vi "Rotate.vi"(8 "error in":errorcluster, 9 "Inverse?":bool, 10 "Orient3d in":refnum<class "Orient3d Class.lvclass">, 11 "Vec3d in":refnum<class "Vec3d Class.lvclass">) -> (0 "error out":errorcluster, 3 "Vec3d out":refnum<class "Vec3d Class.lvclass">)   [LabVIEW 2011, in "Vec3d Class.lvclass"]
uses:
  Vec3d Class.lvclass
  Orient3d Class/Orient3d Class.lvclass
  Vec3d Class.lvclass/Vec3d Class.ctl
  <vilib>/Analysis/baseanly.llb/Real A x B.vi
  <vilib>/Analysis/NI_AALBase.lvlib
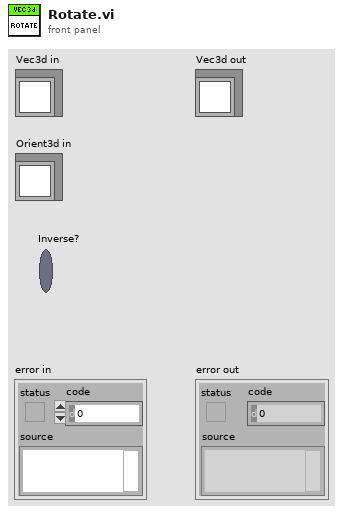
[diagram p1: front panel]
types:
  T1 = typedef "NI_Matrix.lvlib/RealMatrix.ctl" = dbl[][]
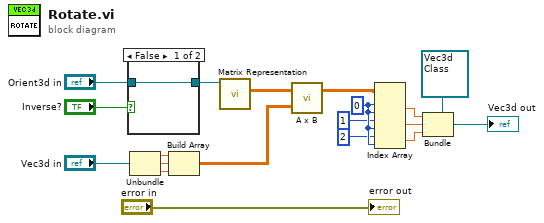
[diagram p0: block diagram]
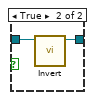
[diagram p2: hidden frame]
diagram:
  w9 = 0 ("index (row)")
  n1 = case shown="False" "Inverse?" {
    tunnel: "Orient3d in" -> [w20 w22]
    tunnel: [w20 w21] -> w16
    frame False {
    }
    frame True {
      n2 = call "Invert.vi"("Orient3d in"=w22) -> ("Orient3d out"=w21:refnum<class "Orient3d Class.lvclass">)  [unwired: 9 in, 1 out]
    }
  }
  n3 = Unbundle("Vec3d in") -> (w15:dbl, w14:dbl, w13:dbl)
  n4 = Build Array(w15, w14, w13) -> (w11:T1)
  n5 = call "Matrix Representation.vi"("Orient3d in"=w16) -> ("Rotation Matrix"=w12:T1)  [unwired: 8 in, 2 out]
  n6 = call-poly <vilib>:"A x B.vi"("B"=w11, "A"=w12) -> ("A x B"=w10:T1)  [unwired: 1 out]
  n7 = Index Array(array=w10, index (row) #1=w9, index (col) #1=w9, index (row) #2=1 ("index (row)"), index (col) #2=w9, index (row) #3=2 ("index (row)"), index (col) #3=w9) -> (element #1=w5:dbl, element #2=w4:dbl, element #3=w3:dbl)
  n8 = Bundle(cluster=refnum<class "Vec3d Class.lvclass"> refnum ("Vec3d out"), w5, w4, w3) -> (→"Vec3d out":refnum<class "Vec3d Class.lvclass">)
  "error out" <- "error in"
